vi "V7310.Message.Get.vi"(6 "timeout ms (5000)":i32=5000, 8 "error in":errorcluster, 11 "Connection in":refnum<k5>) -> (0 "error out":errorcluster, 2 "Messages":T1[](array[typedef]), 3 "Connection out":refnum<k5>)   [LabVIEW 2016]
uses:
  LowLevel/V7310.Message.Data.ctl
  LowLevel/V7310.Commands.ctl
  LowLevel/V7310.Global.vi
panel:
  out "Data out":string
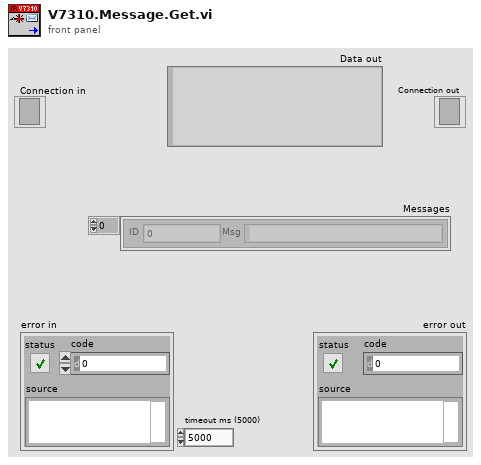
[diagram p1: front panel]
types:
  T1 = typedef "V7310.Message.Data.ctl" = cluster{"ID":i32, "Msg":string}
  T2 = typedef "V7310.Commands.ctl" = enum16{"Start", "Stop", "GetStatus", "GetVarNames", "GetJobNames", "SetJob", "GetJob", "SetVars", "GetVars", "SetLayoutPosition", "SetRotation", "GetMessageID", "GetMessages", "ConfirmMessages", "DeleteMessages", "SetRTC", "GetRTC", "SetVarPosition", "SetIntensity", "GetIntensity", "SetStartTriggerDelay", "GetStartTriggerDelay", "SetStopTriggerDelay", "GetStopTriggerDelay", "SetConsecutiveTriggerDelay", "GetConsecutiveTriggerDelay", "SetMarkSpeed", "GetMarkSpeed"}
  T3 = typedef "V7310.ErrorLevels.ctl" = enum16{"OK", "Warning", "Error"}
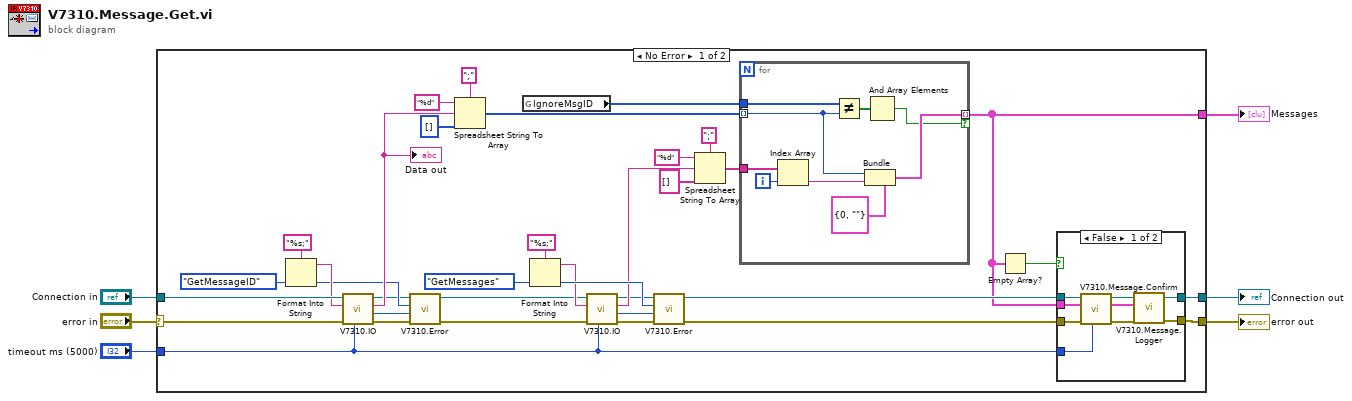
[diagram p0: block diagram]
diagram:
  n1 = case shown="No Error" "error in" {
    selector: "error in" -> [w37 w57]
    tunnel: "Connection in" -> [w38 w58]
    tunnel: [w12 w58] -> w5
    tunnel: "timeout ms (5000)" -> [w9 _]
    tunnel: [w11 w57] -> w2
    tunnel: [w8 _] -> w1
    frame No Error {
      w25 = V7310.Commands."GetMessages" ("Cmd")
      w30 = V7310.Commands."GetMessageID" ("Cmd")
      n2 = Format Into String(format string="%s;", w30) -> (resulting string=w31:string)  [unwired: 2 in, 1 out]
      n3 = call "V7310.IO.vi"("timeout ms (5000)"=w9, "error in"=w37, "Data in"=w31, "Connection in"=w38) -> ("error out"=w28:errorcluster, "Error Level"=w29:T3, "Data out"=w33:string, "Connection out"=w22:refnum<k5>)  [unwired: 4 in]
      "Data out" <- w33
      n4 = call "V7310.Error.vi"("error in"=w28, "Error Level"=w29, "Cmd"=w30) -> ("error out"=w21:errorcluster)  [unwired: 8 in]
      n5 = Spreadsheet String To Array(delimiter (Tab)=";", format string="%d", spreadsheet string=w33, array type (2D Dbl)=i32[] [] ("StrArray")) -> (array=w15:i32[])
      n6 = global read "V7310.Global.vi" "IgnoreMsgID"() -> (w14:i32[])
      n7 = Format Into String(format string="%s;", w25) -> (resulting string=w24:string)  [unwired: 2 in, 1 out]
      n8 = call "V7310.IO.vi"("timeout ms (5000)"=w9, "error in"=w21, "Data in"=w24, "Connection in"=w22) -> ("error out"=w27:errorcluster, "Error Level"=w26:T3, "Data out"=w17:string, "Connection out"=w13:refnum<k5>)  [unwired: 4 in]
      n9 = call "V7310.Error.vi"("error in"=w27, "Error Level"=w26, "Cmd"=w25) -> ("error out"=w10:errorcluster)  [unwired: 8 in]
      n10 = Spreadsheet String To Array(delimiter (Tab)=";", format string="%d", spreadsheet string=w17, array type (2D Dbl)=string[] [] ("StrArray")) -> (array=w16:string[])
      n11 = for {
        tunnel: w16 -> [w55]
        tunnel: w15 -> [w51] mode=indexing
        tunnel: [w56] -> w8 mode=indexing if=w49
        tunnel: w14 -> [w52]
        i -> [w53]
        n12 = Index Array(array=w55, index=w53) -> (element=w54:string)
        n13 = Not Equal?(x=w52, y=w51) -> (x != y?=w50:bool[])
        n14 = Bundle(cluster=T1 {"ID"=0, "Msg"=""} ("Error"), "ID"=w51, "Msg"=w54) -> (w56:T1)
        n15 = And Array Elements(Boolean array=w50) -> (logical AND=w49:bool)
      }
      n16 = Empty Array?(array=w8) -> (empty?=w7:bool)
      n17 = case shown="False" w7 {
        tunnel: w13 -> [w44 w46]
        tunnel: [w43 w46] -> w12
        tunnel: [w42 w47] -> w11
        tunnel: w10 -> [w41 w47]
        tunnel: w9 -> [w40 _]
        tunnel: w8 -> [w39 _]
        frame False {
          n18 = call "V7310.Message.Confirm.vi"("timeout ms (5000)"=w40, "error in"=w41, "Connection in"=w44) -> ("error out"=w45:errorcluster, "Connection out"=w43:refnum<k5>)  [unwired: 7 in]
          n19 = call "V7310.Message.Logger.vi"("error in"=w45, "Messages"=w39) -> ("error out"=w42:errorcluster)  [unwired: 9 in]
        }
        frame True {
        }
      }
    }
    frame Error {
    }
  }
  "Connection out" <- w5
  "error out" <- w2
  "Messages" <- w1
